vi "CreateTargetPath.vi"(0 "Target Path In":path, 5 "Error In":errorcluster) -> (14 "Target Path Out":path, 19 "Error Out":errorcluster)   [LabVIEW 2019]
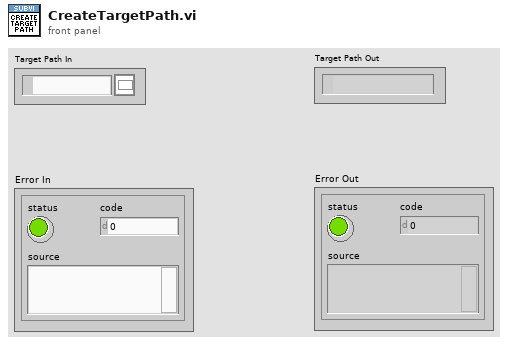
[diagram p1: front panel]
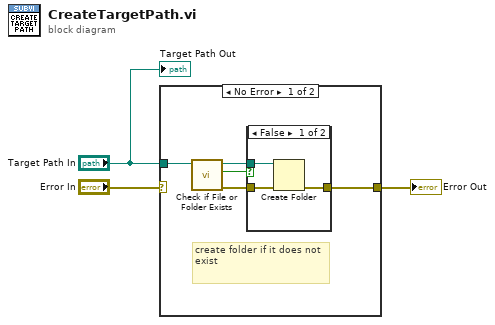
[diagram p0: block diagram]
diagram:
  n1 = case shown="No Error" "Error In" {
    selector: "Error In" -> [_ w13]
    tunnel: "Target Path In" -> [w7 _]
    tunnel: [w8 w13] -> w2
    frame No Error {
      # "create folder if it does not exist"
      n2 = call <vilib>:"Check if File or Folder Exists.vi"("path"=w7) -> ("error out"=w4:errorcluster, "file or folder exists?"=w6:bool, "dup path"=w5:path)  [unwired: 8 in]
      n3 = case shown="False" w6 {
        tunnel: w5 -> [w10 _]
        tunnel: w4 -> [w11 w12]
        tunnel: [w9 w12] -> w8
        frame False {
          n4 = Create Folder(path (use dialog)=w10, error in=w11) -> (error out=w9:errorcluster)  [unwired: 1 in, 2 out]
        }
        frame True {
        }
      }
    }
    frame Error {
    }
  }
  "Error Out" <- w2
  "Target Path Out" <- "Target Path In"
